vi "Read configuration.vi"(7 "force loading?":bool=TRUE, 8 "error in (no error)":errorcluster, 11 "Template in":refnum<class "Template.lvclass">) -> (0 "error out":errorcluster, 3 "Template out":refnum<class "Template.lvclass">)   [LabVIEW 2012, in "Template.lvclass"]
doc: "Reads the XML-based configuration file and populates the configuration cluster accordingly. Configuration file name is <component ID>.xml."
uses:
  Template.lvclass
  <vilib>/Distrio/Murmex/Murmex/Murmex.lvclass
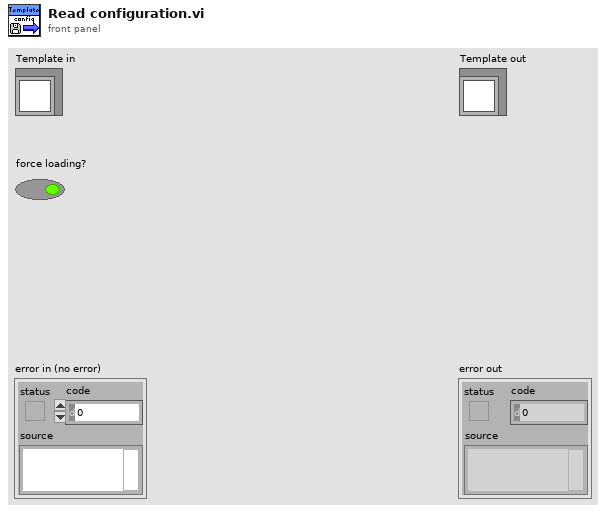
[diagram p1: front panel]
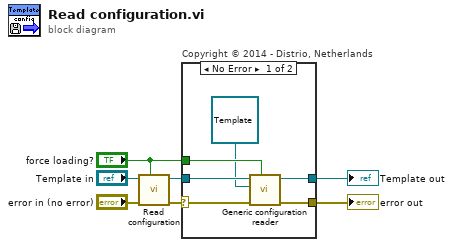
[diagram p0: block diagram]
diagram:
  n1 = call-parent "Read configuration.vi"("force loading?"="force loading?", "error in (no error)"="error in (no error)", "Murmex in"="Template in") -> ("error out"=w5:errorcluster, "Murmex out"=w4:refnum<class "Template.lvclass">)  [unwired: 7 in]
  n2 = case "Copyright © 2014 - Distrio, Netherlands" shown="No Error" w5 {
    selector: w5 -> [w12 w15]
    tunnel: [w8 w15] -> w3
    tunnel: [w9 w14] -> w2
    tunnel: w4 -> [w11 w14]
    tunnel: "force loading?" -> [w13 _]
    frame No Error {
      n3 = call <vilib>:"Generic configuration reader.vi"("force loading?"=w13, "error in (no error)"=w12, "inheritance level"=refnum<class "Template.lvclass"> refnum ("Template.lvclass"), "Murmex in"=w11) -> ("error out"=w8:errorcluster, "Murmex out"=w9:refnum<class "Template.lvclass">)  [unwired: 5 in, 1 out]
    }
    frame Error {
    }
  }
  "error out" <- w3
  "Template out" <- w2
